vi "NotifyIcon - Create SubMenuItem.vi"(8 "error in":errorcluster, 9 "lookup string":string, 10 "MenuItem references":refnum<k24>[](array[refnum]), 11 "SubMenu Title":string) -> (0 "error out":errorcluster, 3 "SubMenuItem reference":refnum<k24>)   [LabVIEW 2015]
uses:
  System.Windows.Forms
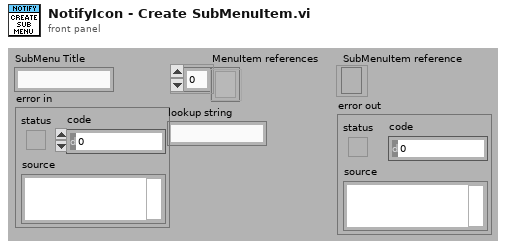
[diagram p1: front panel]
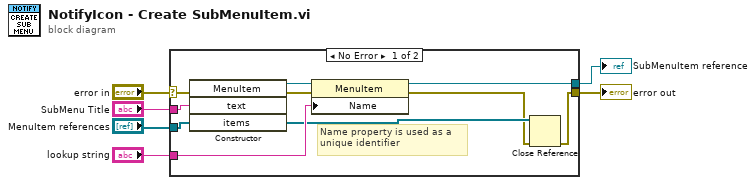
[diagram p0: block diagram]
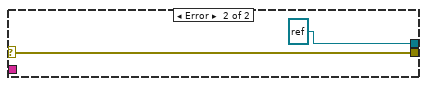
[diagram p2: hidden frame]
diagram:
  n1 = case shown="No Error" "error in" {
    selector: "error in" -> [w10 w18]
    tunnel: "MenuItem references" -> [w16 _]
    tunnel: [w14 refnum<k24> refnum ("new reference")] -> w5
    tunnel: [w7 w18] -> w4
    tunnel: "SubMenu Title" -> [w12 _]
    tunnel: "lookup string" -> [w11 _]
    frame No Error {
      # "Name property is used as a \nunique identifier"
      n2 = constructor class="MenuItem"(error in=w10, "text"=w12, "items"=w16) -> (reference out=w15:refnum<k24>, error out=w13:errorcluster, "items"=w9:refnum<k24>[])  [unwired: 2 in, 2 out]
      n3 = property class="MenuItem"(reference=w15, error in=w13, "Name"=w11) -> (reference out=w14:refnum<k24>, error out=w8:errorcluster)
      n4 = Close Reference(reference=w9, error in (no error)=w8) -> (error out=w7:errorcluster)
    }
    frame Error {
    }
  }
  "error out" <- w4
  "SubMenuItem reference" <- w5
